vi "calculator with sm replicate.vi"() -> ()   [LabVIEW 2020]
panel:
  out "String":string
  in  "Cluster":T1
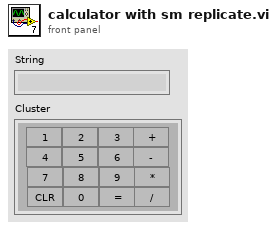
[diagram p1: front panel]
types:
  T1 = cluster{"1":bool, "2":bool, "3":bool, "4":bool, "5":bool, "6":bool, "4 2":bool, "5 2":bool, "6 2":bool, "3 2":bool, "6 3":bool, "6 4":bool, "4 3":bool, "5 3":bool, "6 5":bool, "6 6":bool}
  T2 = enum16{"No Function", "Add", "Subtract", "Multiply", "Divide"}
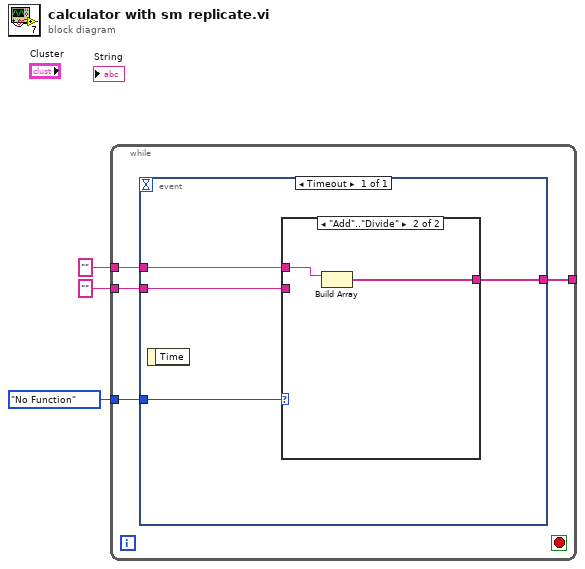
[diagram p0: block diagram]
diagram:
  n1 = while {
    tunnel: "" -> [w7]
    tunnel: "" -> [w6]
    tunnel: T2."No Function" -> [w5]
    tunnel: [w4] -> _
    stop <- _ stop-if-true
    n2 = event shown="[0] Timeout" {
      selector: _ -> [_]
      dyn-events: _ -> [_]
      timeout: _ -> [_]
      tunnel: w7 -> [w11]
      tunnel: w6 -> [w10]
      tunnel: w5 -> [w9]
      tunnel: [w8] -> w4
      event Timeout {
        n3 = event-data() -> ()  [unwired: 1 in, 1 out]
        n4 = case shown="\"Add\"..\"Divide\"" w9 {
          tunnel: w11 -> [_ w13]
          tunnel: w10 -> [_ _]
          tunnel: [_ w12] -> w8
          frame "No Function", Default {
          }
          frame "Add".."Divide" {
            n5 = Build Array(w13) -> (w12:string[])  [unwired: 1 in]
          }
        }
      }
    }
  }
